vi "Start UI.vi"(8 "error in (no error)":errorcluster, 11 "Measurement UI in":refnum<class "Measurement UI.lvclass">) -> (0 "error out":errorcluster, 3 "Measurement UI out":refnum<class "Measurement UI.lvclass">)   [LabVIEW 2017, in "Measurement UI.lvlib" / "Measurement UI.lvclass"]
uses:
  Measurement UI.lvclass
  C:/Program Files (x86)/National Instruments/LabVIEW 2017/vi.lib/ActorFramework/Actor/Actor.lvclass
  <vilib>/ActorFramework/Actor/Actor.lvclass/Actor.ctl
  <vilib>/ActorFramework/Actor/Actor.lvclass
  Controller/Messages/Populate Mesaurements in UI/Display Measurements Message.lvclass
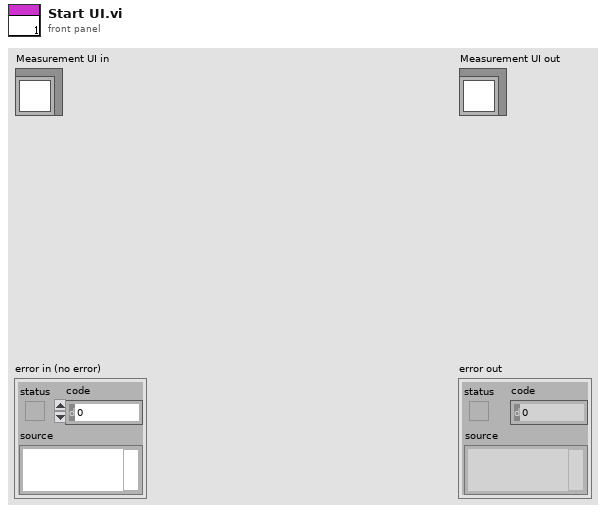
[diagram p1: front panel]
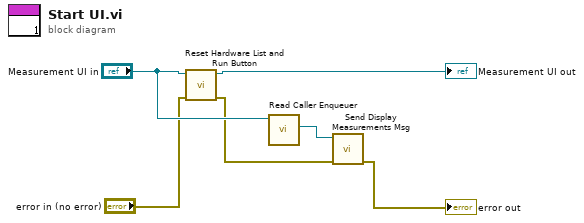
[diagram p0: block diagram]
diagram:
  n1 = call "Reset Hardware List and Run Button.vi"("error in (no error)"="error in (no error)", "Measurement UI in"="Measurement UI in") -> ("error out"=w1:errorcluster, "Measurement UI out"=→"Measurement UI out":refnum<class "Measurement UI.lvclass">)  [unwired: 8 in]
  n2 = call <vilib>:"Read Caller Enqueuer.vi"("Actor"="Measurement UI in") -> ("Caller Enqueuer"=w6:refnum<class "Message Enqueuer.lvclass">)  [unwired: 10 in]
  n3 = call "Send Display Measurements Msg.vi"("error in (no error)"=w1, "Message Enqueuer in"=w6) -> ("error out"=→"error out":errorcluster)  [unwired: 8 in, 1 out]
